vi "ReversedEngineering CheckStateStringTransation.vi"(1 "SelStrings":string[](array[string]), 2 "StringConstant":string) -> (15 "Found":bool, 16 "Index":i32)   [LabVIEW 2012]
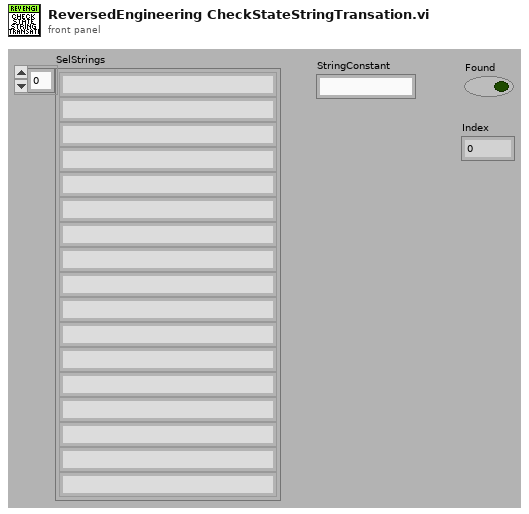
[diagram p1: front panel]
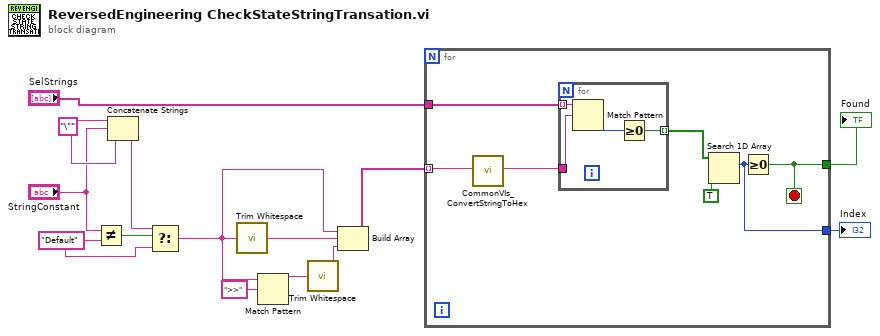
[diagram p0: block diagram]
diagram:
  w9 = "Default" ("y")
  w14 = "\"" ("string")
  n1 = Not Equal?(x="StringConstant", y=w9) -> (x != y?=w10:bool)
  n2 = Concatenate Strings(w14, "StringConstant", w14) -> (w8:string)
  n3 = Select(t=w8, s=w10, f=w9) -> (s? t:f=w6:string)
  n4 = call <vilib>:"Trim Whitespace.vi"("string"=w6) -> ("trimmed string"=w7:string)  [unwired: 1 in]
  n5 = Match Pattern(string=w6, regular expression=">>") -> (before substring=w4:string)  [unwired: 1 in, 3 out]
  n6 = call <vilib>:"Trim Whitespace.vi"("string"=w4) -> ("trimmed string"=w3:string)  [unwired: 1 in]
  n7 = Build Array(w6, w7, w3) -> (w2:string[])
  n8 = for {
    tunnel: [w16] -> w13
    tunnel: "SelStrings" -> [w18]
    tunnel: w2 -> [w17] mode=indexing
    tunnel: [w15] -> w1
    stop <- w16 stop-if-true
    n9 = call <resource>:"CommonVIs_ConvertStringToHex.vi"("inputString"=w17) -> ("outputString"=w21:string)  [unwired: 1 in, 17 out]
    n10 = for {
      tunnel: w18 -> [w25] mode=indexing
      tunnel: [w23] -> w19 mode=indexing
      tunnel: w21 -> [w22]
      n11 = Match Pattern(string=w25, regular expression=w22) -> (offset past match=w24:i32)  [unwired: 4 out]
      n12 = Greater Or Equal To 0?(x=w24) -> (x >= 0?=w23:bool)
    }
    n13 = Search 1D Array(1D array=w19, element=TRUE) -> (index of element=w15:i32)  [unwired: 1 out]
    n14 = Greater Or Equal To 0?(x=w15) -> (x >= 0?=w16:bool)
  }
  "Found" <- w13
  "Index" <- w1
